vi "Remove ans Stop Panel.vi"(8 "error in (no error)":errorcluster, 10 "Index":i32, 11 "Item_Refnums_Array":T1[](array[typedef])) -> (0 "error out":errorcluster, 3 "Item_Refnums_Array Out":T1[](array[typedef]))   [LabVIEW 2013, in "UI Panels.lvlib" / "Panels_XControl.xctl"]
uses:
  Panels_XControl.xctl
  Controls/References/Panel_Refnums.ctl
  Controls/Panel_Command_Enum.ctl
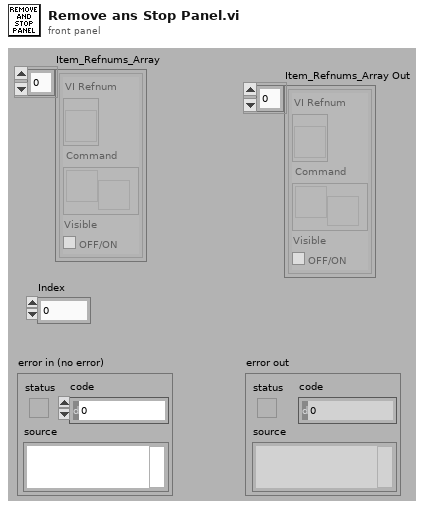
[diagram p1: front panel]
types:
  T1 = typedef "UI Panels.lvlib/Panels_XControl.xctl/Panel_Refnums.ctl" = cluster{"VI Refnum":refnum<vi>, "Command":refnum<user-event>, "Visible":bool}
  T2 = typedef "UI Panels.lvlib/Panels_XControl.xctl/Panel_Command_Enum.ctl" = enum16{"Idle", "Remove & Stop", "Add Item", "Delete Item", "Delete All", "Insert into Subpanel", "Register Menu Events", "Update Value", "Remove from Subpanel", "Set Title", "Set Menu Items", "Insert SubPanel", "Set Splitter Position", "Set Splitter Properties", "Add Menu Items"}
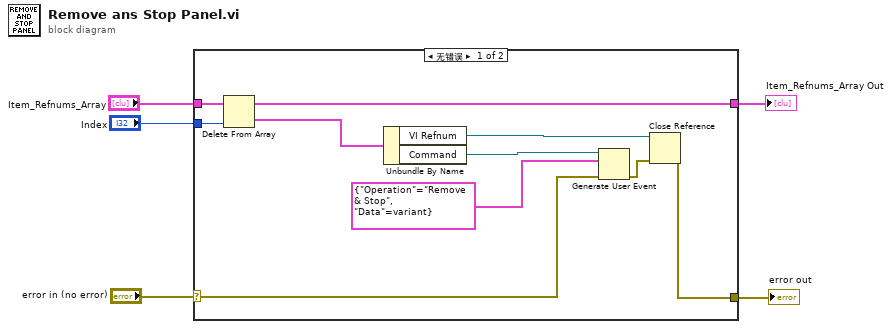
[diagram p0: block diagram]
diagram:
  n1 = case shown="无错误" "error in (no error)" {
    selector: "error in (no error)" -> [w7 w16]
    tunnel: [w13 w16] -> w5
    tunnel: "Index" -> [w12 _]
    tunnel: "Item_Refnums_Array" -> [w11 w17]
    tunnel: [w10 w17] -> w2
    frame No Error {
      n2 = Delete From Array "Delete From Array"(array=w11, index=w12) -> (deleted portion=w14:T1, array with subset deleted=w10:T1[])  [unwired: 1 in]
      n3 = Unbundle By Name(w14) -> ("VI Refnum"=w15:refnum<vi>, "Command"=w9:refnum<user-event>)
      n4 = Generate User Event(user event=w9, event data cluster=cluster{"Operation":T2, "Data":variant} {"Operation"=enum."Remove & Stop", "Data"=variant} ("Item_Command"), error in=w7) -> (error out=w8:errorcluster)  [unwired: 1 in, 1 out]
      n5 = Close Reference(reference=w15, error in (no error)=w8) -> (error out=w13:errorcluster)
    }
    frame Error {
    }
  }
  "Item_Refnums_Array Out" <- w2
  "error out" <- w5
